vi "Parse Multipart Upload Parameters.vi"(11 "Multipart Upload Parameters":T1) -> (3 "HTTP Headers":T4[](array[typedef]))   [LabVIEW 2015, in "NI_AWS_S3.lvlib"]
uses:
  NI_AWS_S3.lvlib
  Core/HTTP Request/Name Value Pair.ctl
  PUT Object Request Parameters.ctl
  ACL.ctl
  Storage Class.ctl
  Core/HTTP Request/HTTP Request.lvclass
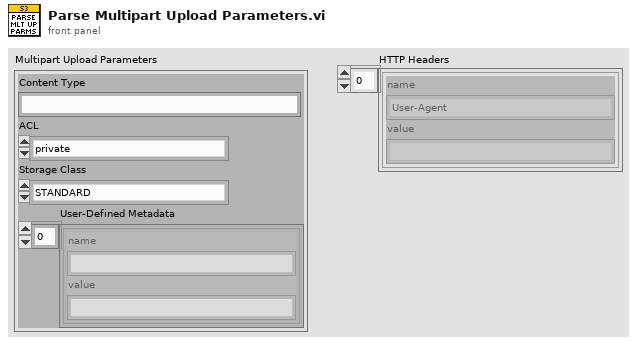
[diagram p1: front panel]
types:
  T1 = typedef "NI_AWS_S3.lvlib/PUT Object Request Parameters.ctl" = cluster{"Content Type":string, "ACL":T2, "Storage Class":T3, "User-Defined Metadata":T4[]}
  T2 = typedef "NI_AWS_S3.lvlib/ACL.ctl" = enum16{"private", "public-read", "public-read-write", "aws-exec-read", "authenticated-read", "bucket-owner-read", "bucket-owner-full-control"}
  T3 = typedef "NI_AWS_S3.lvlib/Storage Class.ctl" = enum16{"STANDARD", "REDUCED_REDUNDANCY"}
  T4 = typedef "NI_AWS_Core.lvlib/HTTP Request.lvclass/Name Value Pair.ctl" = cluster{"name":string, "value":string}
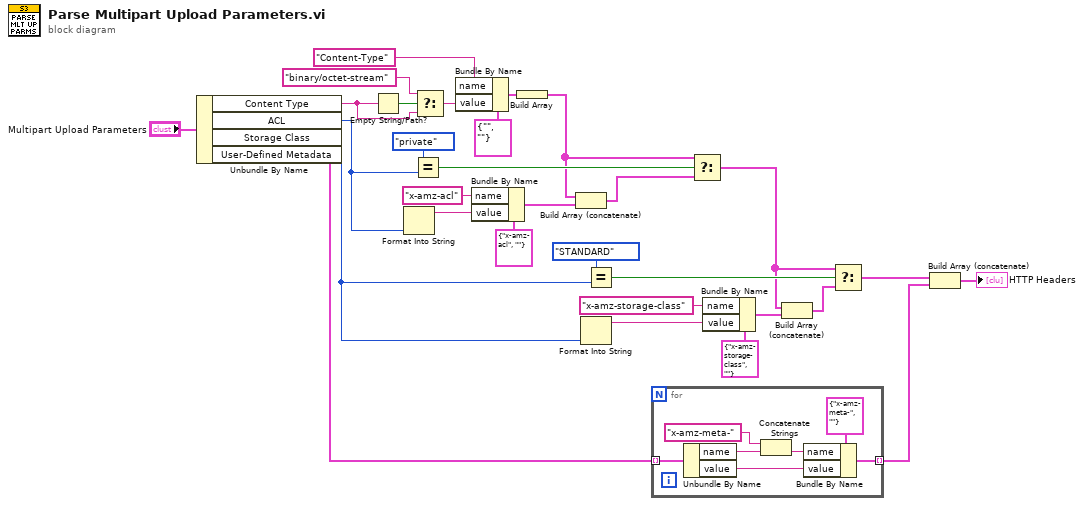
[diagram p0: block diagram]
diagram:
  n1 = Unbundle By Name("Multipart Upload Parameters") -> ("Content Type"=w13:string, "ACL"=w5:T2, "Storage Class"=w4:T3, "User-Defined Metadata"=w1:T4[])
  n2 = Empty String/Path?(string/path=w13) -> (empty?=w14:bool)
  n3 = Format Into String(w5) -> (resulting string=w26:string)  [unwired: 3 in, 1 out]
  n4 = Equal?(x=ACL."private" ("ACL"), y=w5) -> (x = y?=w29:bool)
  n5 = Select(t="binary/octet-stream", s=w14, f=w13) -> (s? t:f=w11:string)
  n6 = Bundle By Name(cluster=T4 {"name"="", "value"=""} ("Name Value Pair"), "name"="Content-Type", "value"=w11) -> (w10:T4)
  n7 = Bundle By Name(cluster=T4 {"name"="x-amz-acl", "value"=""} ("Name Value Pair"), "name"="x-amz-acl", "value"=w26) -> (w25:T4)
  n8 = Build Array(w10) -> (w9:T4[])
  n9 = Build Array (concatenate)(w9, w25) -> (w28:T4[])
  n10 = Format Into String(w4) -> (resulting string=w23:string)  [unwired: 3 in, 1 out]
  n11 = Equal?(x=Storage_Class."STANDARD" ("Storage Class"), y=w4) -> (x = y?=w20:bool)
  n12 = for {
    tunnel: w1 -> [w37] mode=indexing
    tunnel: [w31] -> w17 mode=indexing
    n13 = Unbundle By Name(w37) -> ("name"=w35:string, "value"=w32:string)
    n14 = Concatenate Strings("x-amz-meta-", w35) -> (w33:string)
    n15 = Bundle By Name(cluster=T4 {"name"="x-amz-meta-", "value"=""} ("Name Value Pair"), "name"=w33, "value"=w32) -> (w31:T4)
  }
  n16 = Select(t=w9, s=w29, f=w28) -> (s? t:f=w19:T4[])
  n17 = Bundle By Name(cluster=T4 {"name"="x-amz-storage-class", "value"=""} ("Name Value Pair"), "name"="x-amz-storage-class", "value"=w23) -> (w24:T4)
  n18 = Build Array (concatenate)(w19, w24) -> (w21:T4[])
  n19 = Select(t=w19, s=w20, f=w21) -> (s? t:f=w15:T4[])
  n20 = Build Array (concatenate)(w15, w17) -> (→"HTTP Headers":T4[])
